vi "dfd_Calculate FIR Direct.vi"(4 "coef idx":T1={"start"=0, "stepsize"=1}, 5 "#taps per phase":i32, 6 "coef":i64[](array[numeric]), 7 "fwl_diff":i16, 9 "state idx":T1={"start"=0, "stepsize"=1}, 10 "state in":i64[](array[numeric])) -> (3 "y":i64)   [LabVIEW 2017, in "NI_DigFilter_FXP.lvlib"]
uses:
  <vilib>/addons/Digital Filter Design/NI_DigFilter_FXP.lvlib
  <vilib>/addons/Digital Filter Design/_Objects.llb/dfd_Index Config.ctl
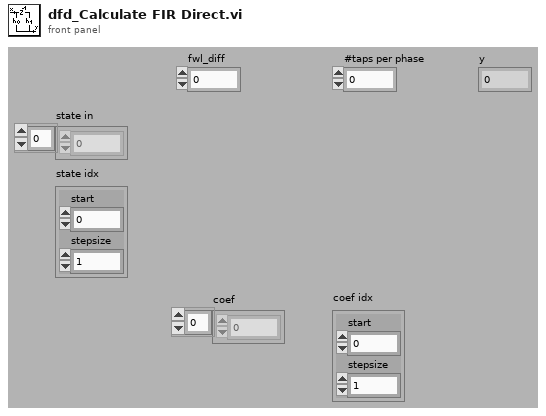
[diagram p1: front panel]
types:
  T1 = typedef "dfd_Index Config.ctl" = cluster{"start":i32, "stepsize":i32}
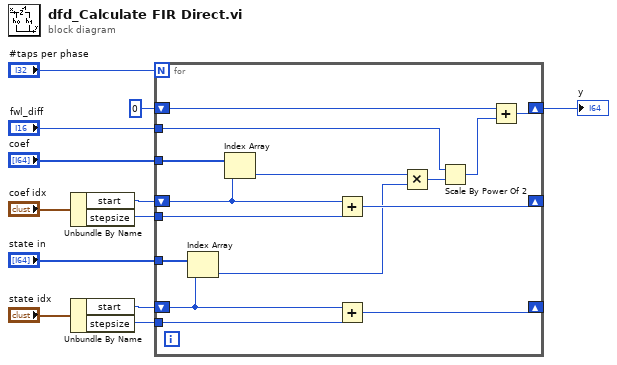
[diagram p0: block diagram]
diagram:
  n1 = Unbundle By Name("coef idx") -> ("start"=w11:i32, "stepsize"=w9:i32)
  n2 = Unbundle By Name("state idx") -> ("start"=w7:i32, "stepsize"=w8:i32)
  n3 = for {
    N: "#taps per phase" -> [_]
    shift-right: [w24] -> _
    shift-left: w11 -> [w26]
    tunnel: "coef" -> [w27]
    tunnel: w9 -> [w25]
    shift-right: [w20] -> _
    shift-left: w7 -> [w22]
    tunnel: w8 -> [w21]
    tunnel: "state in" -> [w23]
    shift-right: [w18] -> w4
    shift-left: i64 0 ("x+y") -> [w19]
    tunnel: "fwl_diff" -> [w13]
    n4 = Index Array(array=w23, index=w22) -> (element=w16:i64)
    n5 = Index Array(array=w27, index=w26) -> (element=w17:i64)
    n6 = Add(x=w26, y=w25) -> (x+y=w24:i32)
    n7 = Add(x=w22, y=w21) -> (x+y=w20:i32)
    n8 = Multiply(x=w17, y=w16) -> (x*y=w15:i64)
    n9 = Scale By Power Of 2(n=w13, x=w15) -> (x*2^n=w14:i64)
    n10 = Add(x=w19, y=w14) -> (x+y=w18:i64)
  }
  "y" <- w4
